vi "VelSimpleEstRobot.vi"(7 "dt":dbl, 10 "Array in":T1[](array[typedef]) {"height" format="%+4.3f"; "pixel_y" format="%+4.3f"; "pixel_x" format="%+4.3f"; "orientation" format="%+4.3f"; "y" format="%+4.3f"; "confidence" format="%4.3f"; "x" format="%+4.3f"}, 11 "Robots Out":T1[](array[typedef]) {"height" format="%+4.3f"; "pixel_y" format="%+4.3f"; "pixel_x" format="%+4.3f"; "orientation" format="%+4.3f"; "y" format="%+4.3f"; "confidence" format="%4.3f"; "x" format="%+4.3f"}) -> (3 "Array out":T1[](array[typedef]) {"height" format="%+4.3f"; "pixel_y" format="%+4.3f"; "pixel_x" format="%+4.3f"; "orientation" format="%+4.3f"; "y" format="%+4.3f"; "confidence" format="%4.3f"; "x" format="%+4.3f"})   [LabVIEW 2018]
uses:
  SSL Detection Robot.ctl
  <vilib>/Analysis/Matrix/Datatypes/RealMatrix.ctl
  <vilib>/Analysis/Matrix/NI_Matrix.lvlib
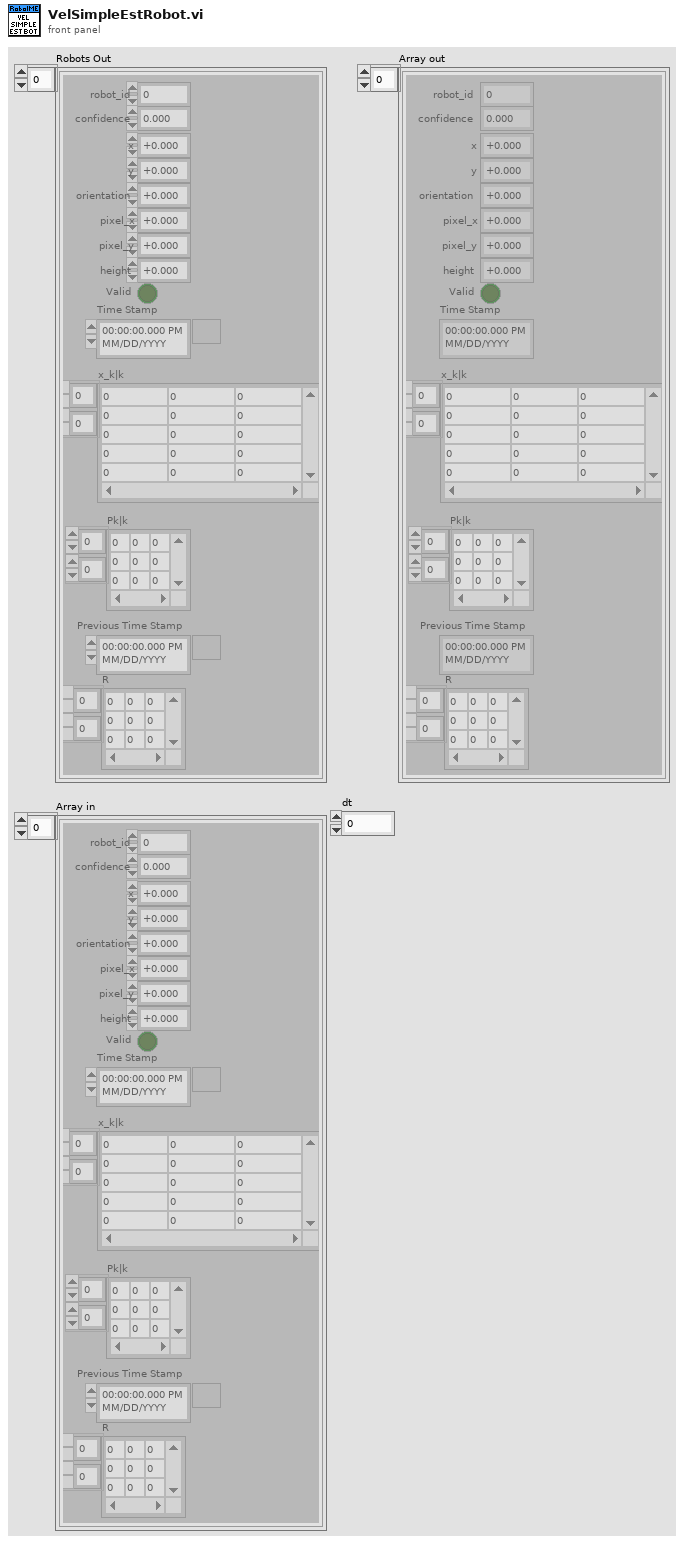
[diagram p1: front panel]
types:
  T1 = typedef "SSL Detection Robot.ctl" = cluster{"x":sgl, "robot_id":u32, "confidence":sgl, "y":sgl, "orientation":sgl, "pixel_x":sgl, "pixel_y":sgl, "height":sgl, "Valid":bool, "Time Stamp":timestamp, "x_k|k":T2, "Pk|k":T2, "Previous Time Stamp":timestamp, "R":T2}
  T2 = typedef "NI_Matrix.lvlib/RealMatrix.ctl" = dbl[][]
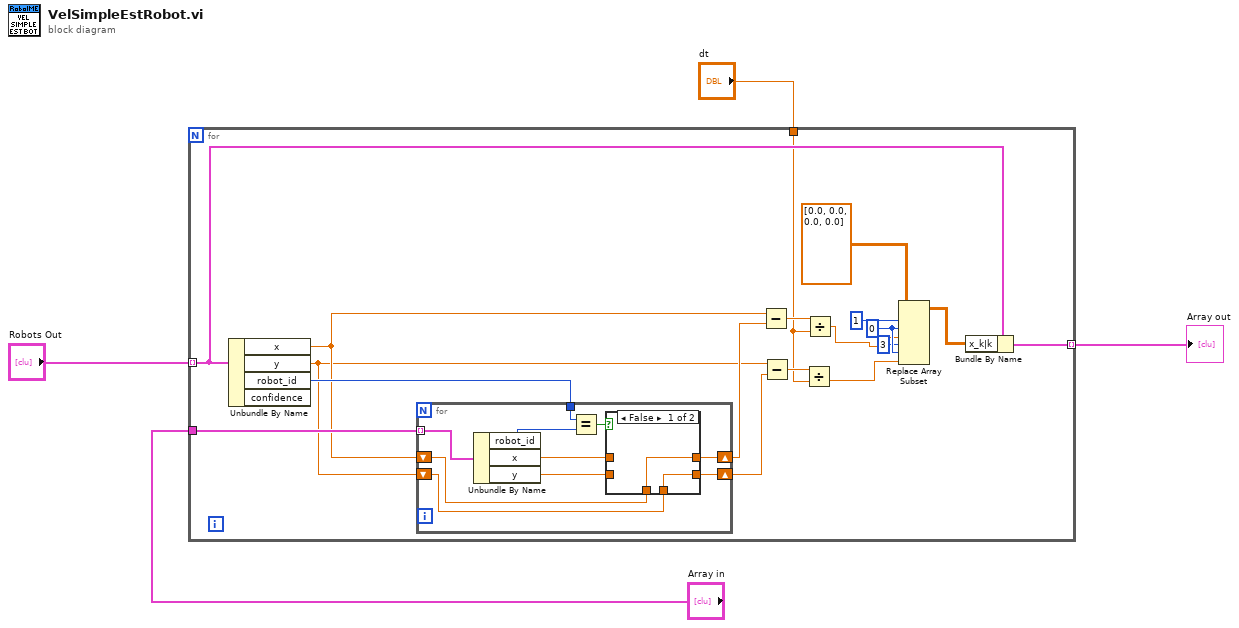
[diagram p0: block diagram]
diagram:
  n1 = for {
    tunnel: "Robots Out" -> [w14] mode=indexing
    tunnel: "Array in" -> [w22]
    tunnel: [w11] -> w3 mode=indexing
    tunnel: "dt" -> [w5]
    w9 = 0 ("disabled index (col)")
    n2 = Unbundle By Name(w14) -> ("x"=w20:sgl, "y"=w18:sgl, "robot_id"=w21:u32)  [unwired: 1 out]
    n3 = for {
      tunnel: w22 -> [w32] mode=indexing
      tunnel: w21 -> [w29]
      shift-right: [w28] -> w19
      shift-left: w20 -> [w24]
      shift-right: [w25] -> w17
      shift-left: w18 -> [w23]
      n4 = Unbundle By Name(w32) -> ("robot_id"=w30:u32, "x"=w27:sgl, "y"=w26:sgl)
      n5 = Equal?(x=w29, y=w30) -> (x = y?=w31:bool)
      n6 = case shown="False" w31 {
        tunnel: [w34 w36] -> w28
        tunnel: w27 -> [_ w36]
        tunnel: [w33 w35] -> w25
        tunnel: w26 -> [_ w35]
        tunnel: w24 -> [w34 _]
        tunnel: w23 -> [w33 _]
        frame False {
        }
        frame True {
        }
      }
    }
    n7 = Subtract(x=w20, y=w19) -> (x-y=w16:sgl)
    n8 = Subtract(x=w18, y=w17) -> (x-y=w15:sgl)
    n9 = Divide(x=w15, y=w5) -> (x/y=w6:dbl)
    n10 = Divide(x=w16, y=w5) -> (x/y=w7:dbl)
    n11 = Replace Array Subset(array=T2 [[0.0], [0.0], [0.0], [0.0]] ("x_k|k"), new element #1=w7, index (row) #1=1 ("index (row)"), index (col) #1=w9, new element #2=w6, index (row) #2=3 ("disabled index (row)"), index (col) #2=w9) -> (w12:T2)
    n12 = Bundle By Name(cluster=w14, "x_k|k"=w12) -> (w11:T1)
  }
  "Array out" <- w3
